vi "Close Session.vi"(8 "error in (no error)":errorcluster, 11 "ApplicationAPI in":refnum<class "TemplateAPI.lvclass">) -> (0 "error out":errorcluster)   [LabVIEW 2018, in "TemplateAPI.lvclass"]
uses:
  TemplateAPI.lvclass
  C:/Users/Phalanx/Documents/LabVIEW-Application-API-Template/Classes/AppControlAPI/AppControlAPI.lvclass
  AppControlAPI/AppControlAPI.lvclass
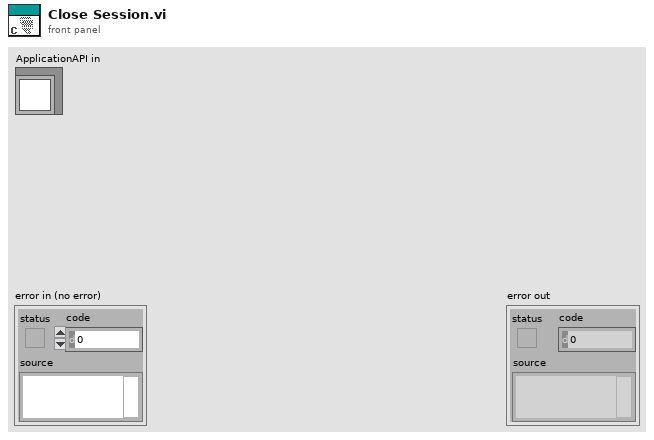
[diagram p1: front panel]
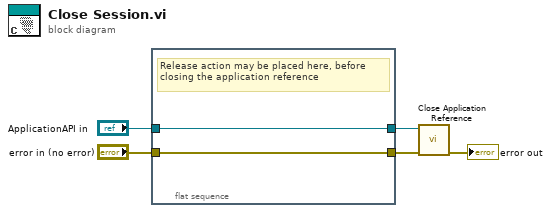
[diagram p0: block diagram]
diagram:
  n1 = flat-sequence {
    tunnel: "error in (no error)" -> [w7]
    tunnel: [w7] -> w2
    tunnel: "ApplicationAPI in" -> [w6]
    tunnel: [w6] -> w3
    frame #0 {
      # "Release action may be placed here, before closing the application reference"
    }
  }
  n2 = call "Close Application Reference.vi"("error in (no error)"=w2, "App Control API in"=w3) -> ("error out"=→"error out":errorcluster)  [unwired: 8 in, 1 out]
